vi "Get Table Path.vi"(8 "error in (no error)":errorcluster, 10 "Table Name":string, 11 "Data.PG":refnum<class "LV-Data.PGSQL.lvclass">) -> (0 "error out":errorcluster, 1 "Exists?":bool, 2 "Table Path":string, 3 "Data.PG out":refnum<class "LV-Data.PGSQL.lvclass">)   [LabVIEW 2019, in "LV-Data.PGSQL.lvclass"]
uses:
  LV-Data.PGSQL.lvclass
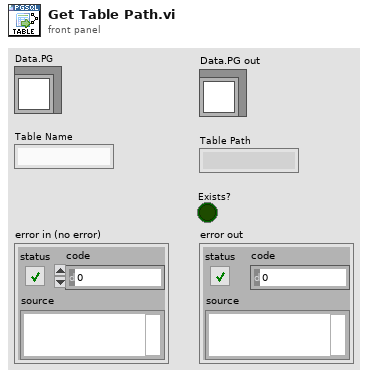
[diagram p1: front panel]
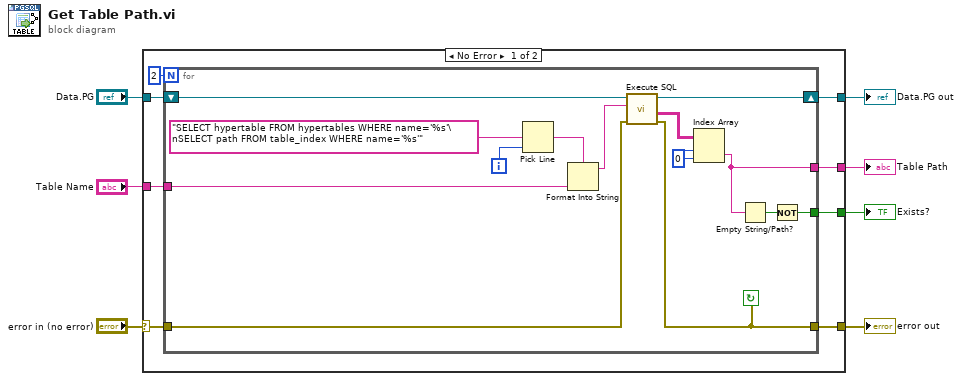
[diagram p0: block diagram]
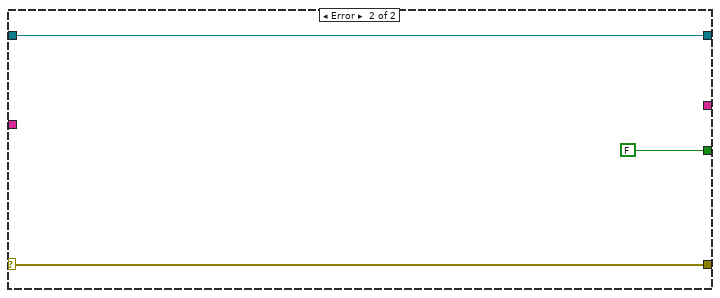
[diagram p2: hidden frame]
diagram:
  n1 = case shown="No Error" "error in (no error)" {
    selector: "error in (no error)" -> [w9 w32]
    tunnel: "Table Name" -> [w15 _]
    tunnel: "Data.PG" -> [w14 w31]
    tunnel: [w13 w32] -> w5
    tunnel: [w12 w31] -> w4
    tunnel: [w11 _] -> w3
    tunnel: [w10 FALSE] -> w2
    frame No Error {
      n2 = for {
        N: 2 -> [_]
        tunnel: w15 -> [w29]
        tunnel: [w25] -> w11
        tunnel: [w23] -> w10
        shift-right: [w26] -> w12
        shift-left: w14 -> [w27]
        tunnel: w9 -> [w22]
        tunnel: [w17] -> w13
        i -> [w19]
        stop <- w17 continue-if-true
        w18 = 0 ("disabled index (col)")
        n3 = Pick Line(multi-line string="SELECT hypertable FROM hypertables WHERE name='%s'\nSELECT path FROM table_index WHERE name='%s'" ("format string"), line index=w19) -> (output string=w20:string)  [unwired: 1 in]
        n4 = Format Into String(format string=w20, w29) -> (resulting string=w28:string)  [unwired: 2 in, 1 out]
        n5 = call "Execute SQL.vi"("error in"=w22, "SQL"=w28, "LV-Data.PGSQL"=w27) -> ("error out"=w17:errorcluster, "Result"=w16:string[][], "LV-Data.PGSQL out"=w26:refnum<class "LV-Data.PGSQL.lvclass">)  [unwired: 5 in, 1 out]
        n6 = Index Array(array=w16, index (row)=w18, index (col)=w18) -> (element=w25:string)
        n7 = Empty String/Path?(string/path=w25) -> (empty?=w24:bool)
        n8 = Not(x=w24) -> (.not. x?=w23:bool)
      }
    }
    frame Error {
    }
  }
  "error out" <- w5
  "Table Path" <- w3
  "Data.PG out" <- w4
  "Exists?" <- w2
